vi "Write Error log file.vi"(8 "error in (no error)":errorcluster, 10 "Error log file":path, 11 "Error Log in":refnum<class "Error Log.lvclass">) -> (0 "error out":errorcluster, 3 "Error Log out":refnum<class "Error Log.lvclass">)   [LabVIEW 2020, in "Error Log.lvclass"]
uses:
  Error Log.lvclass
  Error Log.lvclass/Error Log.ctl
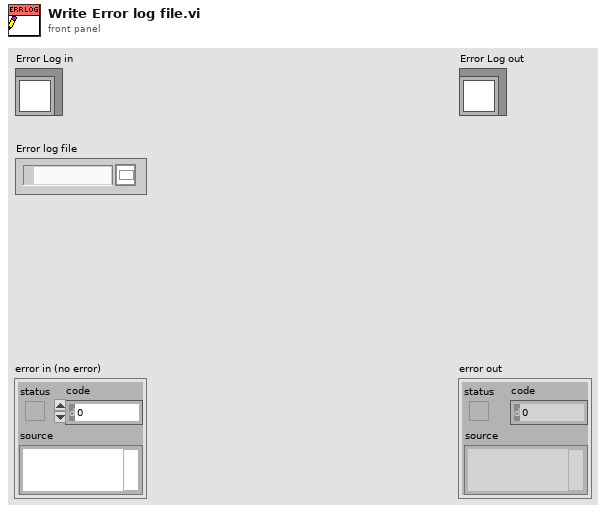
[diagram p1: front panel]
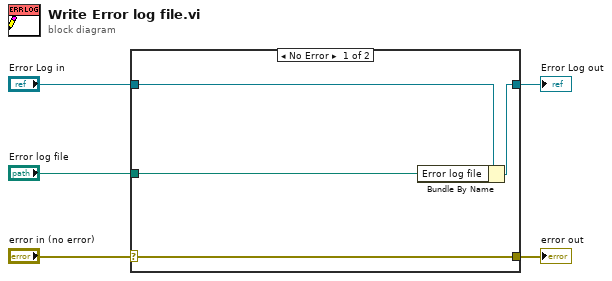
[diagram p0: block diagram]
diagram:
  n1 = case shown="No Error" "error in (no error)" {
    selector: "error in (no error)" -> [w9 w10]
    tunnel: [w9 w10] -> w4
    tunnel: [w7 w11] -> w2
    tunnel: "Error Log in" -> [w8 w11]
    tunnel: "Error log file" -> [w6 _]
    frame No Error {
      n2 = Bundle By Name(cluster=w8, "Error log file"=w6) -> (w7:refnum<class "Error Log.lvclass">)
    }
    frame Error {
    }
  }
  "error out" <- w4
  "Error Log out" <- w2
